vi "pp2_DAQinit.vi"(8 "error in (no error)":errorcluster, 11 "Daq config in":T1={"Sound AO"="Dev2/ao0", "Shock intesity AO"="Dev1/ao1", "Code/LED DO"="Dev1/port1:2", "Switches DI"="Dev1/port0/line0:1", "Webcam"="cam0", "Sound AO task"="", "Sound card task"=0, "Shock intensity AO task"="", "Code/LED DO task"="", "Switch DI task"="", "AO <=> Sound card"=FALSE, "Sound card"=0, "sample rate"=8000.0, "Variable shock"=FALSE, "Webcam on"=FALSE, "Tone gate PFI"="/Dev1/PFI1", "Waveform memo"={"t0"=timestamp(0 s since 1904-01-01), "dt"=1.0, "Y"=[]}} {"sample rate" min=8000.0; "Sound card task" format="%.0x"}) -> (0 "error out":errorcluster, 3 "Daq config out":T1={"Sound AO"="Dev2/ao0", "Shock intesity AO"="Dev1/ao1", "Code/LED DO"="Dev1/port1:2", "Switches DI"="Dev1/port0/line0:1", "Webcam"="cam0", "Sound AO task"="", "Sound card task"=0, "Shock intensity AO task"="", "Code/LED DO task"="", "Switch DI task"="", "AO <=> Sound card"=FALSE, "Sound card"=0, "sample rate"=8000.0, "Variable shock"=FALSE, "Webcam on"=FALSE, "Tone gate PFI"="/Dev1/PFI1", "Waveform memo"={"t0"=timestamp(0 s since 1904-01-01), "dt"=1.0, "Y"=[]}} {"sample rate" min=8000.0; "Sound card task" format="%.0x"})   [LabVIEW 2013]
uses:
  pp2_CTL_DaqConfig.ctl
  <vilib>/userdefined/High Color/IMAQdx.ctl
  <vilib>/sound2/lvsound2.llb/Sound Output Task ID.ctl
  <vilib>/sound2/lvsound2.llb/Sampling Mode.ctl
  <vilib>/sound2/lvsound2.llb/Sound Data Format.ctl
  <vilib>/DAQmx/create/channels.llb/DAQmx Create Channel (DO-Digital Output).vi
  <vilib>/DAQmx/create/channels.llb/DAQmx Create Channel (AO-Voltage-Basic).vi
  <vilib>/DAQmx/configure/timing.llb/DAQmx Timing (Sample Clock).vi
  <resource>/objmgr/daqmx.rc
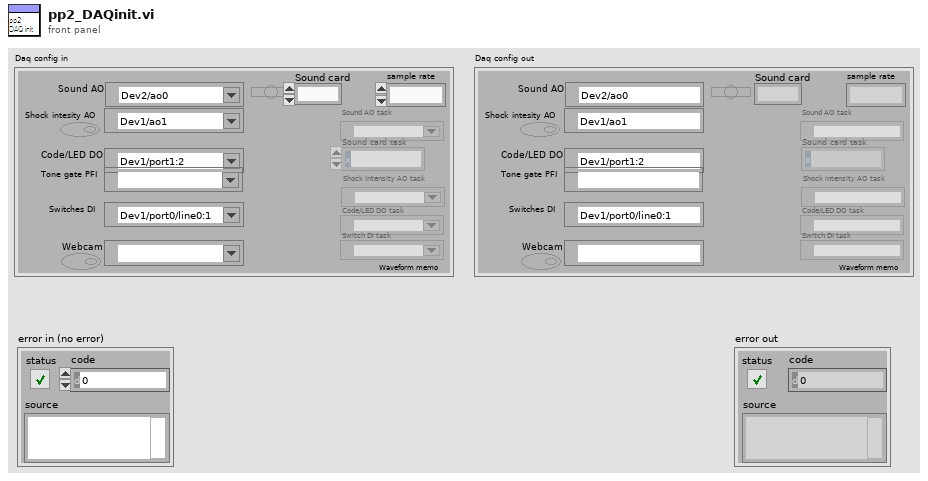
[diagram p1: front panel]
types:
  T1 = typedef "pp2_CTL_DaqConfig.ctl" = cluster{"Sound AO":tag, "Shock intesity AO":tag, "Code/LED DO":tag, "Switches DI":tag, "Webcam":T2, "Sound AO task":refnum<k21>, "Sound card task":T3, "Shock intensity AO task":refnum<k21>, "Code/LED DO task":refnum<k21>, "Switch DI task":refnum<k21>, "AO <=> Sound card":bool, "Sound card":u32, "sample rate":dbl, "Variable shock":bool, "Webcam on":bool, "Tone gate PFI":tag, "Waveform memo":waveform(dbl)}
  T2 = typedef "IMAQdx.ctl" = refnum<k21>
  T3 = typedef "Sound Output Task ID.ctl" = u32
  T4 = typedef "Sound Data Format.ctl" = cluster{"sample rate (S/s)":dbl, "number of channels":i32, "bits per sample":i32}
  T5 = typedef "Sampling Mode.ctl" = i32
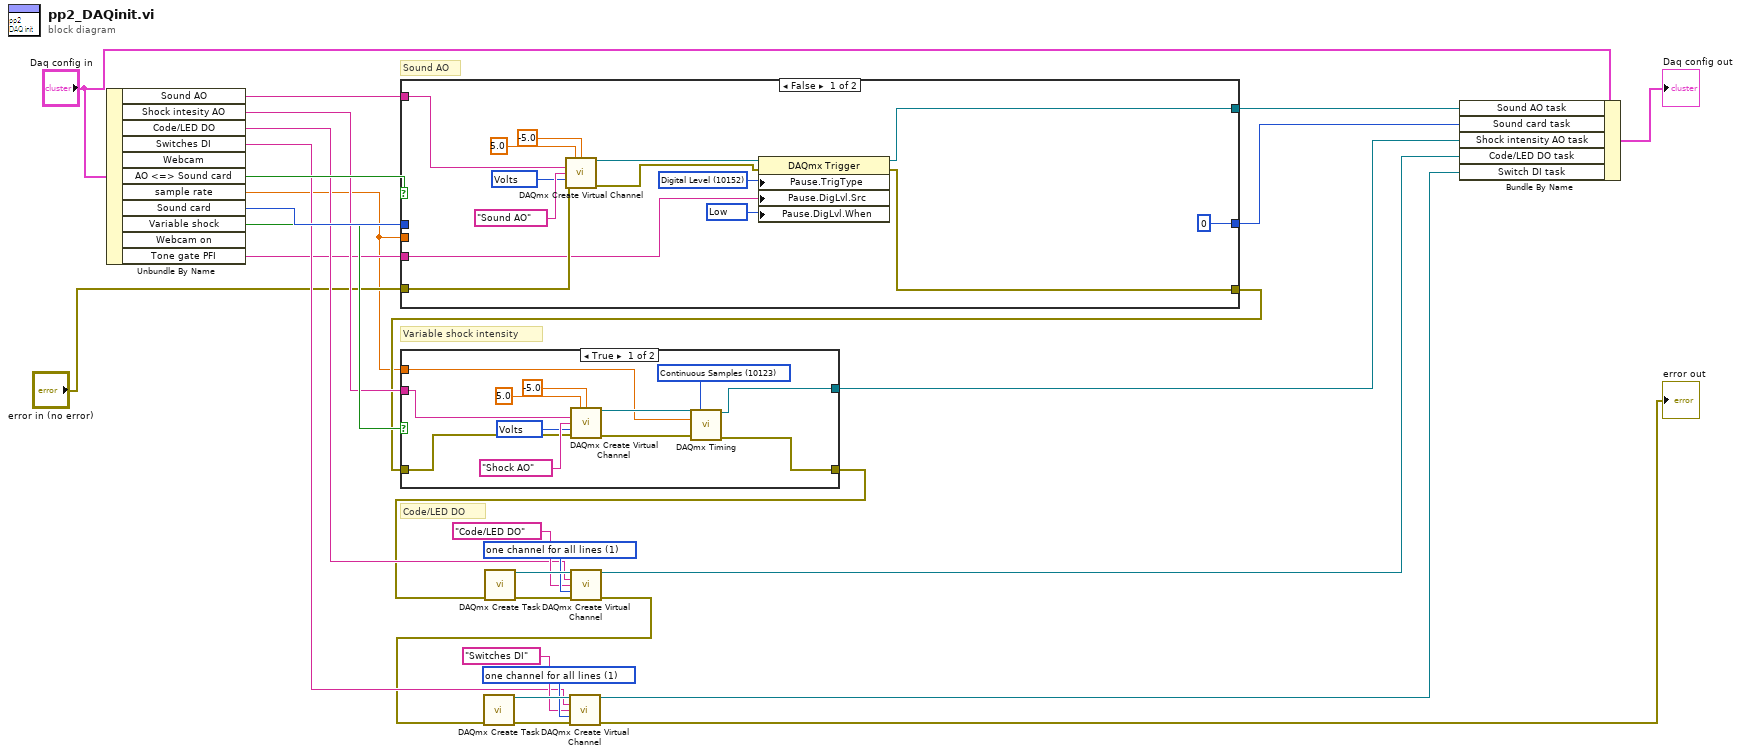
[diagram p0: block diagram]
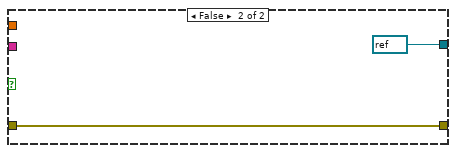
[diagram p2: hidden frame]
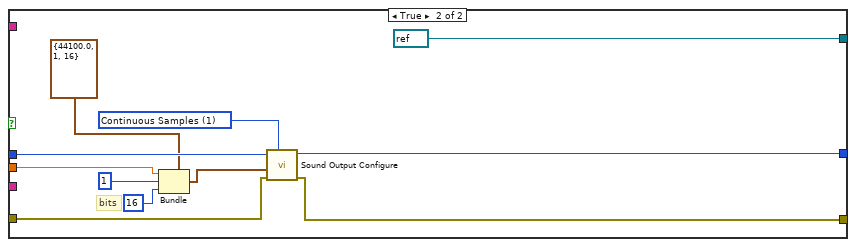
[diagram p3: hidden frame]
diagram:
  w12 = 1 items=["one channel for each line", "one channel for all lines"] ("line grouping")
  w17 = 1 items=["one channel for each line", "one channel for all lines"] ("line grouping")
  # "Code/LED DO"
  # "Variable shock intensity"
  # "Sound AO"
  n1 = Unbundle By Name("Daq config in") -> ("Sound AO"=w28:tag, "Shock intesity AO"=w21:tag, "Code/LED DO"=w15:tag, "Switches DI"=w10:tag, "AO <=> Sound card"=w29:bool, "sample rate"=w1:dbl, "Sound card"=w24:u32, "Variable shock"=w22:bool, "Tone gate PFI"=w2:tag)  [unwired: 2 out]
  n2 = case shown="False" w29 {
    tunnel: w28 -> [w43 _]
    tunnel: [w33 refnum<k21> refnum ("task out")] -> w25
    tunnel: w24 -> [_ w53]
    tunnel: [T3 0 ("task ID") w49] -> w23
    tunnel: "error in (no error)" -> [w37 w48]
    tunnel: [w31 w47] -> w6
    tunnel: w2 -> [w32 _]
    tunnel: w1 -> [_ w46]
    frame False {
      w35 = 10214 items=["High"=10192, "Low"=10214] ("Pause.DigLvl.When")
      w36 = 10152 items=["Analog Level"=10101, "Analog Window"=10103, "Digital Level"=10152, "Digital Pattern"=10398, "None"=10230] ("Pause.TrigType")
      w39 = 10348 items=["Volts"=10348, "From Custom Scale"=10065] ("units")
      n3 = call-poly <vilib>:"DAQmx Create Virtual Channel.vi"("maximum value"=5.0, "minimum value"=-5.0, "physical channels"=w43, "name to assign"="Sound AO", "units"=w39, "error in"=w37) -> ("task out"=w34:refnum<k21>, "error out"=w30:errorcluster)  [unwired: 8 in]
      n4 = property class="DAQmx Trigger"(reference=w34, error in=w30, "Pause.TrigType"=w36, "Pause.DigLvl.Src"=w32, "Pause.DigLvl.When"=w35) -> (reference out=w33:refnum<k21>, error out=w31:errorcluster)
    }
    frame True {
      w52 = T5 1 items=["Finite Samples", "Continuous Samples"] ("sample mode")
      # "bits"
      n5 = Bundle(cluster=T4 {"sample rate (S/s)"=44100.0, "number of channels"=1, "bits per sample"=16} ("sound format"), "sample rate (S/s)"=w46, "number of channels"=1 ("Input.BufSize"), "bits per sample"=16 ("Input.BufSize")) -> (w44:T4)
      n6 = call <vilib>:"Sound Output Configure.vi"("sample mode"=w52, "error in (no error)"=w48, "sound format"=w44, "device ID"=w53) -> ("error out"=w47:errorcluster, "task ID"=w49:T3)  [unwired: 6 in]
    }
  }
  n7 = case shown="True" w22 {
    tunnel: w21 -> [w63 _]
    tunnel: [w59 refnum<k21> refnum ("task out")] -> w20
    tunnel: w1 -> [w58 _]
    tunnel: w6 -> [w57 w67]
    tunnel: [w56 w67] -> w5
    frame True {
      w55 = 10123 items=["Finite Samples"=10178, "Continuous Samples"=10123, "Hardware Timed Single Point"=12522] ("sample mode")
      w64 = 10348 items=["Volts"=10348, "From Custom Scale"=10065] ("units")
      n8 = call-poly <vilib>:"DAQmx Create Virtual Channel.vi"("maximum value"=5.0, "minimum value"=-5.0, "physical channels"=w63, "name to assign"="Shock AO", "units"=w64, "error in"=w57) -> ("task out"=w61:refnum<k21>, "error out"=w60:errorcluster)  [unwired: 8 in]
      n9 = call-poly <vilib>:"DAQmx Timing.vi"("task/channels in"=w61, "sample mode"=w55, "rate"=w58, "error in"=w60) -> ("task out"=w59:refnum<k21>, "error out"=w56:errorcluster)  [unwired: 10 in]
    }
    frame False {
    }
  }
  n10 = call <vilib>:"DAQmx Create Task.vi"("error in"=w5) -> ("task out"=w18:refnum<k21>, "error out"=w19:errorcluster)  [unwired: 13 in]
  n11 = call-poly <vilib>:"DAQmx Create Virtual Channel.vi"("task in"=w18, "lines"=w15, "name to assign"="Code/LED DO", "line grouping"=w17, "error in"=w19) -> ("task out"=w9:refnum<k21>, "error out"=w4:errorcluster)  [unwired: 9 in]
  n12 = call <vilib>:"DAQmx Create Task.vi"("error in"=w4) -> ("task out"=w13:refnum<k21>, "error out"=w14:errorcluster)  [unwired: 13 in]
  n13 = call-poly <vilib>:"DAQmx Create Virtual Channel.vi"("task in"=w13, "lines"=w10, "name to assign"="Switches DI", "line grouping"=w12, "error in"=w14) -> ("task out"=w8:refnum<k21>, "error out"=→"error out":errorcluster)  [unwired: 9 in]
  n14 = Bundle By Name(cluster="Daq config in", "Sound AO task"=w25, "Sound card task"=w23, "Shock intensity AO task"=w20, "Code/LED DO task"=w9, "Switch DI task"=w8) -> (→"Daq config out":T1)
